vi "simx Get Last Errors.vi"(7 "operationMode":i32, 8 "error in (no error)":errorcluster, 9 "errorStrings":string, 10 "errorCnt":i32, 11 "clientID":i32) -> (0 "error out":errorcluster, 1 "errorStrings out":string, 2 "errorCnt out":i32, 3 "function return":i32)   [LabVIEW 2019, in "PXL_V-REP.lvlib"]
doc: "EXTAPI_DLLEXPORT simxInt simxGetLastErrors(simxInt clientID,simxInt* errorCnt,simxChar** errorStrings,simxInt operationMode);"
uses:
  PXL_V-REP.lvlib
  <userlib>/V-REP/remoteApi.dll
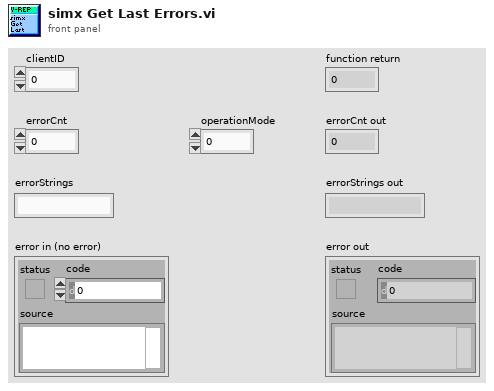
[diagram p1: front panel]
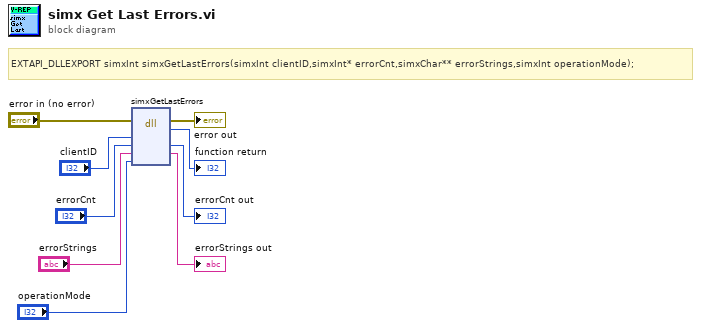
[diagram p0: block diagram]
diagram:
  # "EXTAPI_DLLEXPORT simxInt simxGetLastErrors(simxInt clientID,simxInt* errorCnt,simxChar** errorStrings,simxInt operationMode);"
  n1 = dll-call lib="C:/Program Files (x86)/National Instruments/LabVIEW 2019/user.lib/V-REP/remoteApi.*" fn="simxGetLastErrors"(error in="error in (no error)", "clientID"="clientID", "errorCnt"="errorCnt", "errorStrings"="errorStrings", "operationMode"="operationMode") -> (error out=→"error out":errorcluster, →"function return":i32, "errorCnt"=→"errorCnt out":i32, "errorStrings"=→"errorStrings out":string)  [unwired: 4 in, 1 out]
